vi "Funcion_Apertura.vi"() -> (1 "PIPE OUT":i32, 2 "PIPE IN":i32, 3 "NDISPOSITIVOS":i32)   [LabVIEW 2016]
uses:
  microchip_solutions_v2013-06-15/USB/Tools/MCHPUSB Custom Driver/Mpusbapi/Dll/Borland_C/mpusbapi.dll
panel:
  in  "error in (no error)":errorcluster
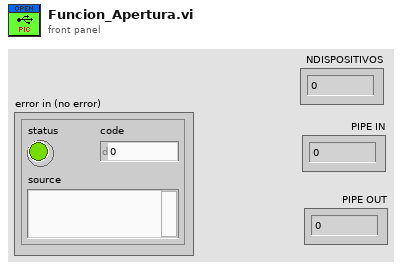
[diagram p1: front panel]
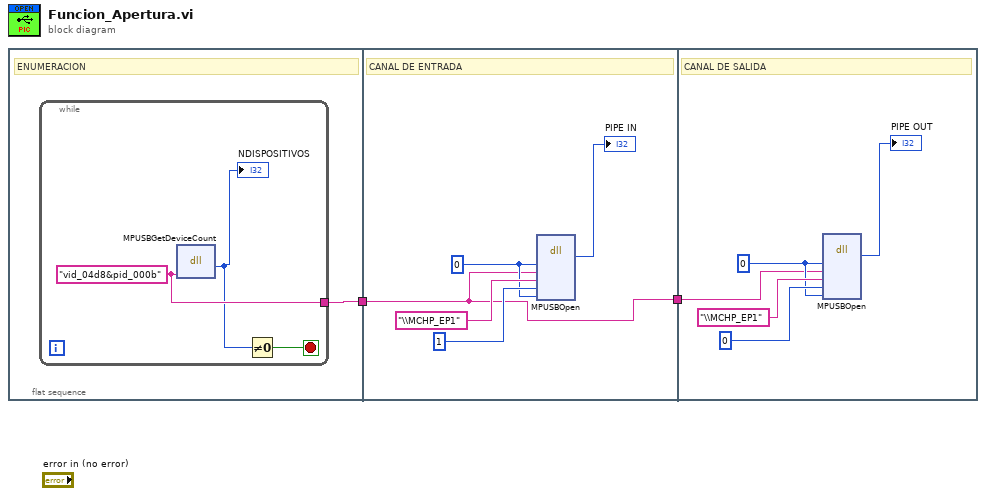
[diagram p0: block diagram]
diagram:
  n1 = flat-sequence {
    tunnel: [w3] -> w2
    tunnel: w2 -> [w7]
    tunnel: [w7] -> w1
    tunnel: w1 -> [w12]
    frame #0 {
      # "ENUMERACION"
      n2 = while {
        tunnel: [w6] -> w3
        stop <- w5 stop-if-true
        w6 = "vid_04d8&pid_000b" ("VID_PID")
        n3 = dll-call lib="C:/microchip_solutions_v2013-06-15/USB/Tools/MCHPUSB Custom Driver/Mpusbapi/Dll/Borland_C/mpusbapi.dll" fn="MPUSBGetDeviceCount"("VID_PID"=w6) -> ("NDISPOSITIVOS"=w4:i32)  [unwired: 4 in, 2 out]
        "NDISPOSITIVOS" <- w4
        n4 = Not Equal To 0?(x=w4) -> (x != 0?=w5:bool)
      }
    }
    frame #1 {
      w8 = 0 ("Instancia")
      # "CANAL DE ENTRADA"
      n5 = dll-call lib="C:/microchip_solutions_v2013-06-15/USB/Tools/MCHPUSB Custom Driver/Mpusbapi/Dll/Borland_C/mpusbapi.dll" fn="MPUSBOpen"("Instancia"=w8, "VID_PID"=w7, "pEP"="\\MCHP_EP1", "dwDIR"=1, "dwReserved"=w8) -> ("PIPE"=→"PIPE IN":i32)  [unwired: 8 in, 2 out]
    }
    frame #2 {
      w13 = 0 ("Instancia")
      # "CANAL DE SALIDA"
      n6 = dll-call lib="C:/microchip_solutions_v2013-06-15/USB/Tools/MCHPUSB Custom Driver/Mpusbapi/Dll/Borland_C/mpusbapi.dll" fn="MPUSBOpen"("Instancia"=w13, "VID_PID"=w12, "pEP"="\\MCHP_EP1", "dwDIR"=0, "dwReserved"=w13) -> ("PIPE"=→"PIPE OUT":i32)  [unwired: 8 in, 2 out]
    }
  }
